vi "Read value.vi"(8 "error in (no error)":errorcluster, 11 "UserDefinedWaveform in":refnum<class "UserDefinedWaveform.lvclass">) -> (0 "error out":errorcluster, 2 "value":cluster{"t0":dbl, "dt":dbl, "y":dbl[]}, 3 "UserDefinedWaveform out":refnum<class "UserDefinedWaveform.lvclass">)   [LabVIEW 2014, in "UserDefinedWaveform.lvclass"]
uses:
  UserDefinedWaveform.lvclass
  UserDefinedWaveform.lvclass/UserDefinedWaveform.ctl
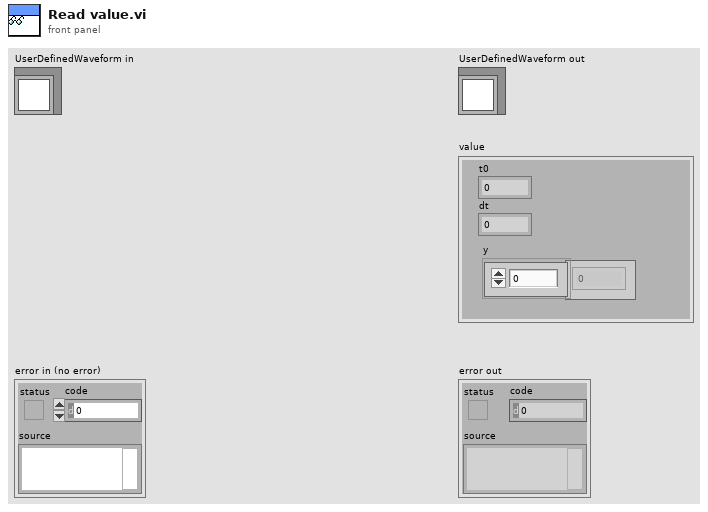
[diagram p1: front panel]
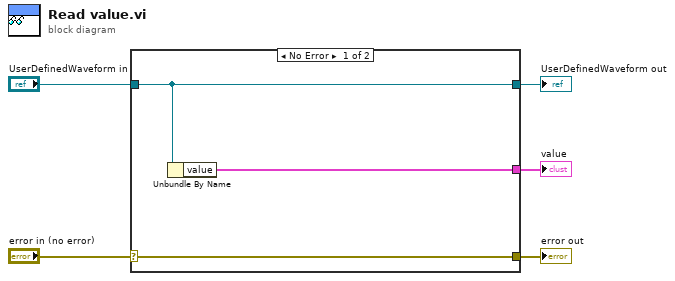
[diagram p0: block diagram]
diagram:
  n1 = case shown="No Error" "error in (no error)" {
    selector: "error in (no error)" -> [w8 w9]
    tunnel: [w8 w9] -> w4
    tunnel: [w7 w10] -> w2
    tunnel: "UserDefinedWaveform in" -> [w7 w10]
    tunnel: [w6 _] -> w1
    frame No Error {
      n2 = Unbundle By Name(w7) -> ("value"=w6:cluster{"t0":dbl, "dt":dbl, "y":dbl[]})
    }
    frame Error {
    }
  }
  "error out" <- w4
  "UserDefinedWaveform out" <- w2
  "value" <- w1
